vi "reset revision history.vi"(6 "Top Level/Always Included VIs":path[](array[path]), 7 "Main Destination Path":path, 9 "Target Name":string, 10 "Build Specification Name":string, 11 "Project Path":path) -> (0 "error out":errorcluster)   [LabVIEW 2019]
panel:
  out "VIs":string[](array[string])
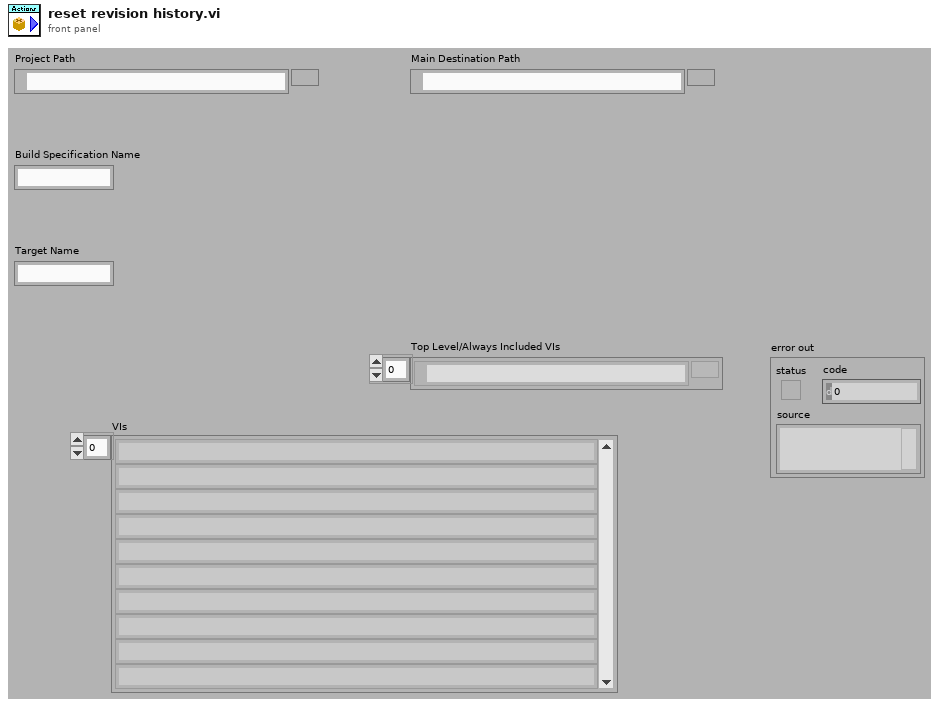
[diagram p1: front panel]
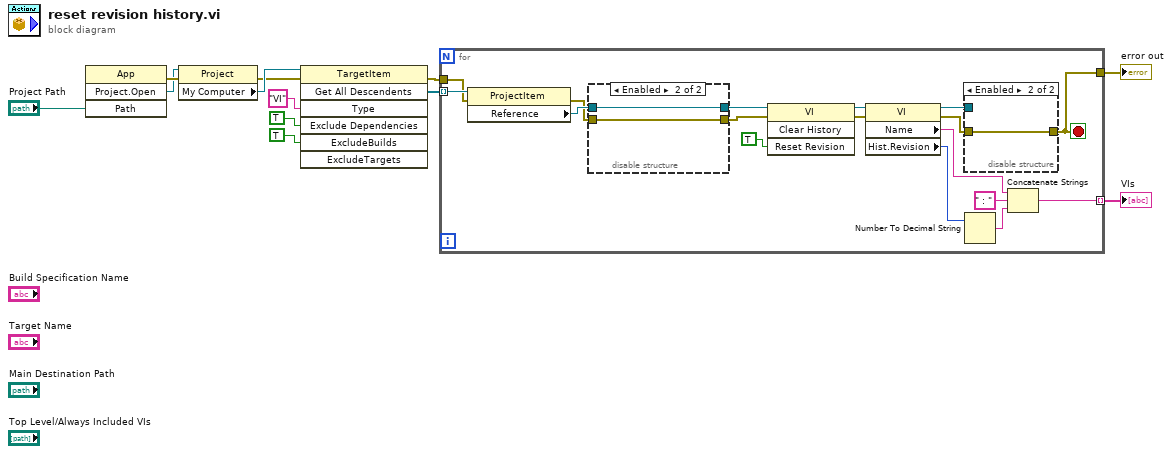
[diagram p0: block diagram]
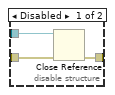
[diagram p2: hidden frame]
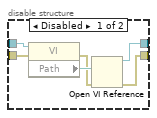
[diagram p3: hidden frame]
diagram:
  n1 = invoke class="App" method="Project.Open"("Path"="Project Path") -> (error out=w11:errorcluster, "Project:Open"=w10:refnum<vi>)  [unwired: 3 in, 2 out]
  n2 = property class="Project"(reference=w10, error in=w11) -> (error out=w6:errorcluster, "My Computer"=w9:refnum<vi>)  [unwired: 1 out]
  n3 = invoke class="TargetItem" method="Get All Descendents"(reference=w9, error in=w6, "Type"="VI", "Exclude Dependencies"=TRUE ("ExcludeDependencies"), "ExcludeBuilds"=TRUE) -> (error out=w5:errorcluster, "All Descendents"=w8:refnum<vi>[])  [unwired: 2 in, 5 out]
  n4 = for {
    tunnel: w8 -> [w29] mode=indexing
    tunnel: w5 -> [w27]
    tunnel: [w19] -> w4
    tunnel: [w15] -> w3 mode=indexing
    stop <- w19 stop-if-true
    n5 = property class="ProjectItem"(reference=w29, error in=w27) -> (error out=w18:errorcluster, "Reference"=w24:refnum<vi>)  [unwired: 1 out]
    n6 = disable-structure shown="Enabled" {
      disable-tunnel: w24 -> [w39 w41]
      disable-tunnel: [w37 w41] -> w23
      disable-tunnel: w18 -> [w36 w40]
      disable-tunnel: [w34 w40] -> w17
      frame Disabled {
        n7 = property on="Property Node" class="VI"(reference=w39, error in=w36) -> (error out=w35:errorcluster, "Path"=w38:path)  [unwired: 1 out]
        n8 = Open VI Reference(vi path=w38, error in (no error)=w35) -> (vi reference=w37:refnum<vi>, error out=w34:errorcluster)  [unwired: 4 in]
      }
      frame Enabled {
      }
    }
    n9 = invoke class="VI" method="Clear History"(reference=w23, error in=w17, "Reset Revision"=TRUE) -> (reference out=w25:refnum<vi>, error out=w21:errorcluster)  [unwired: 1 in, 2 out]
    n10 = property class="VI"(reference=w25, error in=w21) -> (reference out=w22:refnum<vi>, error out=w20:errorcluster, "Name"=w14:string, "Hist.Revision"=w26:u32)
    n11 = disable-structure shown="Enabled" {
      disable-tunnel: w22 -> [w32 _]
      disable-tunnel: w20 -> [w31 w33]
      disable-tunnel: [w30 w33] -> w19
      frame Disabled {
        n12 = Close Reference(reference=w32, error in (no error)=w31) -> (error out=w30:errorcluster)
      }
      frame Enabled {
      }
    }
    n13 = Number To Decimal String(number=w26) -> (decimal integer string=w16:string)  [unwired: 1 in]
    n14 = Concatenate Strings(w14, " : " ("string"), w16) -> (w15:string)
  }
  "error out" <- w4
  "VIs" <- w3
